vi "dust type.vi"(0 "Enable":bool=TRUE, 1 "Small?":bool, 5 "error in (no error)":errorcluster) -> (14 "Cancel 2":bool caption="Cancel", 15 "output cluster 2":T2 {"Batch" step=1; "Type" step=1; "Dust Source Builder:" items=["Keith Drake", "Nick Beaty", "Anthony Shu", "David James"]}, 16 "Dust Properties 2":T1, 18 "OK":bool, 19 "error out":errorcluster)   [LabVIEW 2012]
doc: "Displays a standard dialog box that prompts users to enter information, such as a user name and password.\n--------------------\n\nThis Express VI is configured as follows:\n\nMessage to Display to the User:Please Enter Experiment Settings Information For Database Storage.\nThe inputs are: \nNumber: Please Enter Group ID\nText Entry Box: Please Enter Tags:\nText Entry Box: Please Enter Experiment Description:"
uses:
  dust type.ctl
  source_builders.ctl
  dust_type_indicator.ctl
  <vilib>/addons/database/Connection.llb/Conn Execute.vi
  <vilib>/addons/database/Recordset.llb/Rec Fetch Recordset Data (R).vi
  <vilib>/addons/database/Recordset.llb/Rec Destroy - Connection.vi
  <userlib>/_OpenG.lib/array/array.llb/Remove Duplicates from 1D Array (String)__ogtk.vi
  <userlib>/_OpenG.lib/array/array.llb/Search 1D Array (String)__ogtk.vi
  <userlib>/_OpenG.lib/array/array.llb/Index 1D Array Elements (I32)__ogtk.vi
  <userlib>/_OpenG.lib/array/array.llb/Conditional Auto-Indexing Tunnel (I32)__ogtk.vi
  <vilib>/addons/database/_DB Variant To Data/Database Variant To Data.xnode
  <vilib>/addons/database/NI_Database_API.lvlib
panel:
  in  "Transfer":bool caption="OK2"
  out "Comments":string[](array[string])
  out "Dust Properties":T1
  out "Dust Names":string[](array[string])
  out "Dust Weights":dbl[](array[numeric])
  out "Sizes":string[](array[string])
  out "Typical Weights":dbl[](array[numeric])
  out "Densities":dbl[](array[numeric])
  out "Batch Nos":i32[](array[numeric])
  out "Dust Types":i32[](array[numeric])
  out "Dust Type Ids":i32[](array[numeric])
  in  "Controls":T2 {"Batch" min=1 max=1 step=1; "Type" min=1 max=2 step=1; "Dust Source Builder:" items=["Keith Drake", "Nick Beaty", "Anthony Shu", "David James"]}
  in  "Create New":bool caption="OK2"
  in  "Cancel":bool
  in  "Update":bool caption="OK1"
  # "Please Enter Dust Information For Storage in the CCLDAS Database."
  # "Dust Information"
  # "Dust Information"
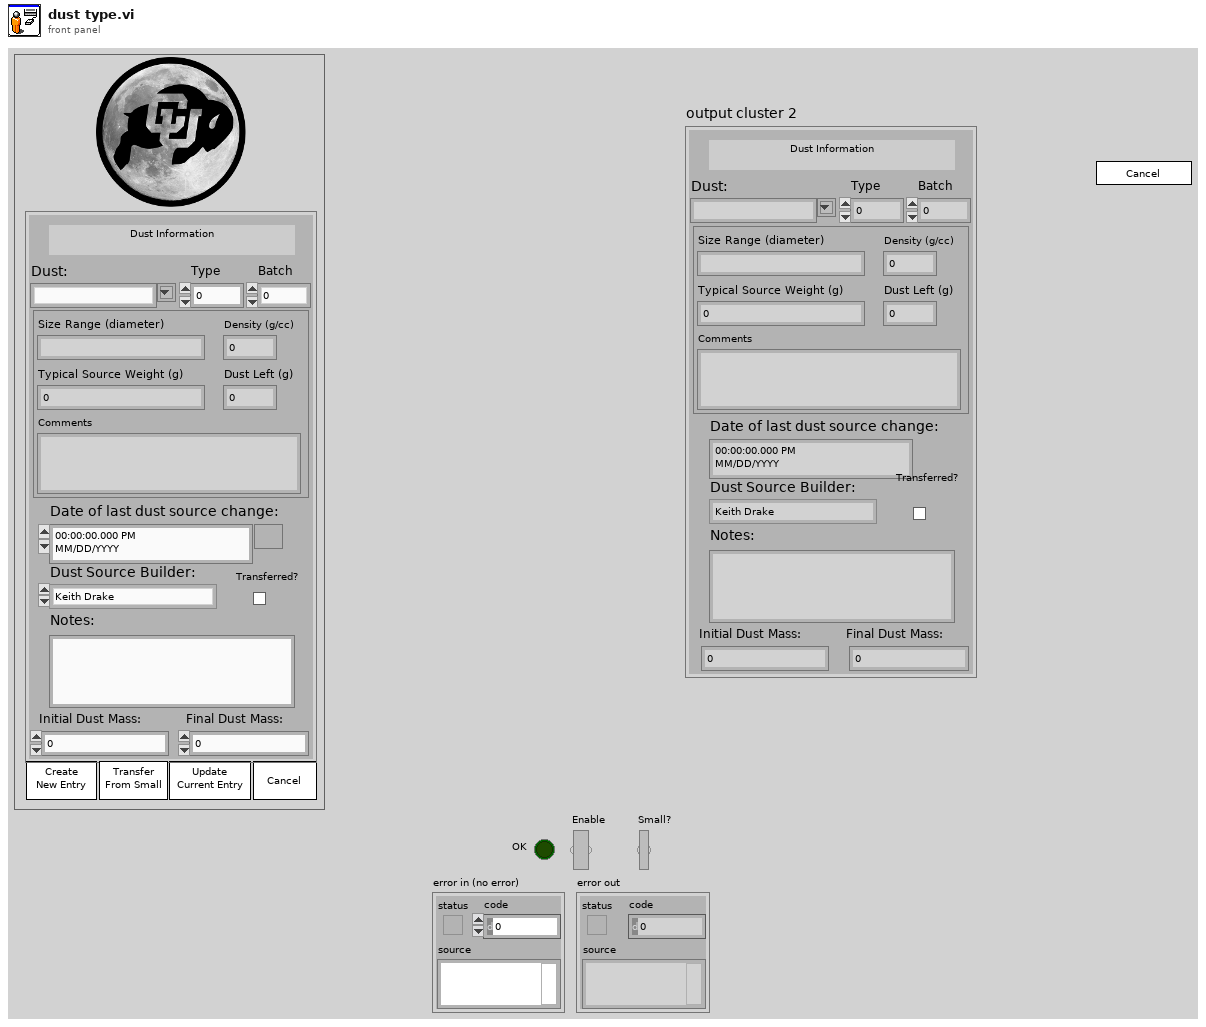
[diagram p1: front panel]
types:
  T1 = typedef "dust_type_indicator.ctl" = cluster{"Size Range (diameter)":string, "Density (g/cc)":dbl, "Typical Source Weight (g)":dbl, "Dust Left (g)":dbl, "Comments":string}
  T2 = typedef "dust type.ctl" = cluster{"Dust info id":u16, "Integer Timestamp":i64, "Dust:":string, "Dust Source Builder:":T3, "Notes:":string, "Date of last dust source change:":timestamp, "Initial Dust Mass:":dbl, "Final Dust Mass:":dbl, "Type":u16, "Batch":u16, "dust type id":u16, "Transferred?":bool}
  T3 = typedef "source_builders.ctl" = u16
  T4 = enum8{"Enabled", "Disabled", "Disabled and Grayed Out"}
  T5 = cluster{"Dust info id":u16, "Integer Timestamp":i64, "dust type id":u16, "Dust Source Builder:":u16, "Notes:":string, "Initial Dust Mass:":dbl, "Final Dust Mass:":dbl, "shot count":u16, "run time":dbl, "From Small\nAccelerator":bool}
  T6 = typedef "NI_Database_API.lvlib/Conn ObjectReference.ctl" = refnum<k1>
  T7 = typedef "NI_Database_API.lvlib/Rec ObjectReference.ctl" = refnum<k1>
  T8 = cluster{"data":string, "data":dbl, "data":dbl, "data":dbl, "data":string}
  T9 = cluster{"Dust event id":dbl, "Integer Time":i64, "dust type id":u16, "Dust Source Builder:":T3, "Notes:":string, "Initial Dust Mass:":dbl, "Dust event id":dbl, "Transferred?":bool}
  T10 = cluster{"Dust event id":dbl, "Integer Time":i64, "dust type id":u16, "Dust Source Builder:":u16, "Notes:":string, "Initial Dust Mass:":dbl, "Final Dust Mass:":dbl, "shot count":u16, "run time":dbl, bool}
  T11 = cluster{"Dust info id":u16, "Integer Timestamp":i64, "dust type id":u16, "Dust Source Builder:":T3, "Notes:":string, "Initial Dust Mass:":dbl, "Final Dust Mass:":dbl, "Transferred?":bool}
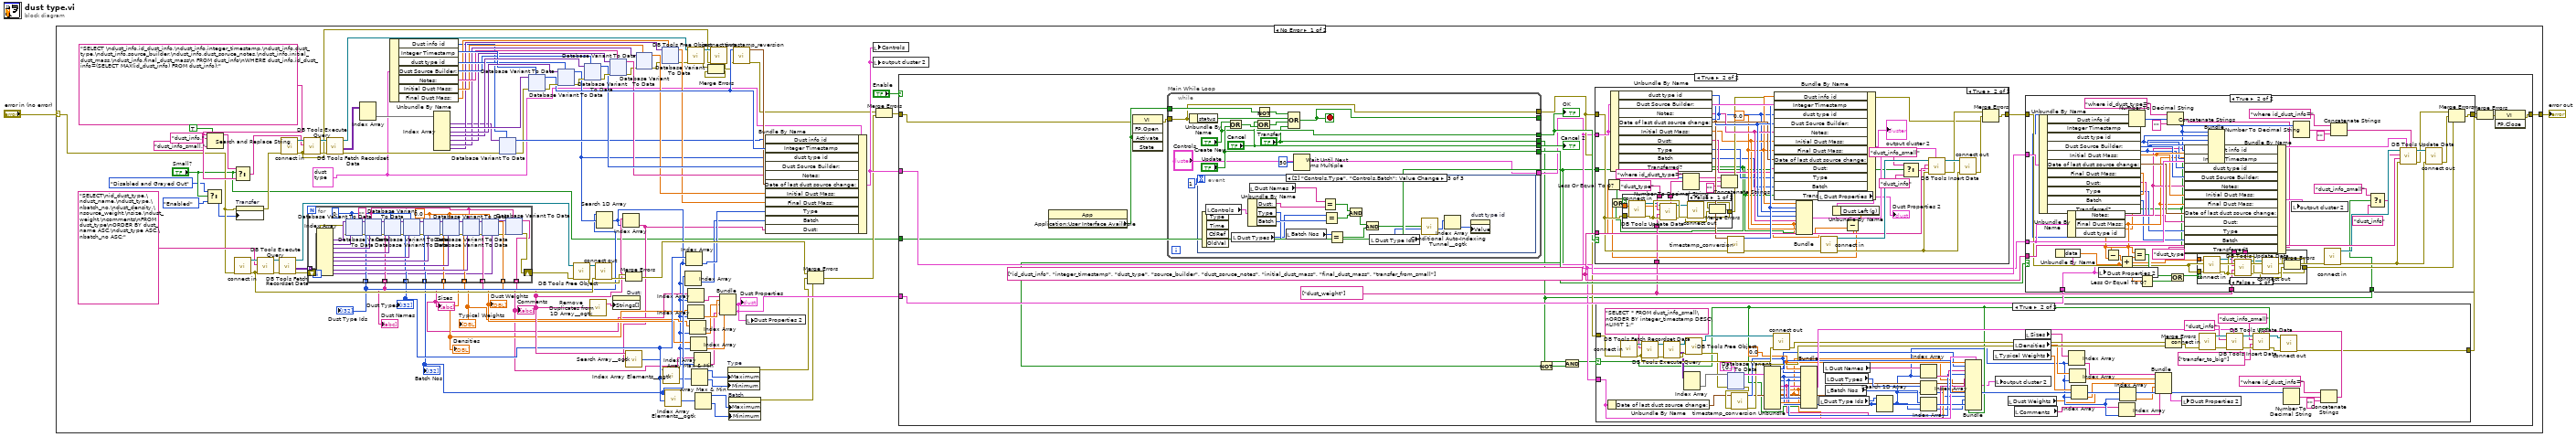
[diagram p0: block diagram]
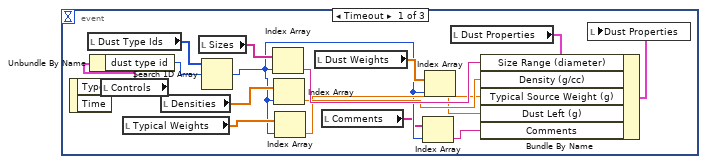
[diagram p6: hidden frame]
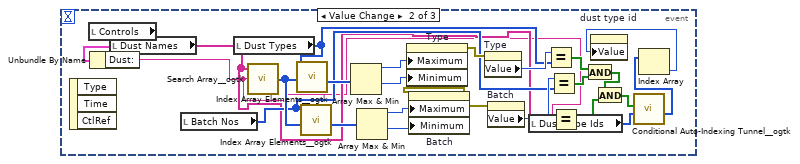
[diagram p7: hidden frame]
diagram:
  n1 = case shown="No Error" "error in (no error)" {
    selector: "error in (no error)" -> [w8 w1234]
    tunnel: [w99 w1234] -> w1
    frame No Error {
      w19 = T2 {"Dust info id"=0, "Integer Timestamp"=0, "Dust:"="", "Dust Source Builder:"=0, "Notes:"="", "Date of last dust source change:"=timestamp(0 s since 1904-01-01), "Initial Dust Mass:"=0.0, "Final Dust Mass:"=0.0, "Type"=0, "Batch"=0, "dust type id"=0, "Transferred?"=FALSE} ("Controls")
      w14 = "SELECT \ndust_info.id_dust_info,\ndust_info.integer_timestamp,\ndust_info.dust_type,\ndust_info.source_builder,\ndust_info.dust_soruce_notes,\ndust_info.initial_dust_mass,\ndust_info.final_dust_mass\n FROM dust_info\nWHERE dust_info.id_dust_info=(SELECT MAX(id_dust_info) FROM dust_info);" ("SQL query")
      n2 = Select(t=T4."Disabled and Grayed Out" ("Disabled"), s="Small?", f=T4."Enabled" ("Disabled")) -> (s? t:f=w3:T4)
      n3 = Search and Replace String(replace all?=TRUE ("replace all? (F)"), input string=w14, search string="dust_info.", replace string="dust_info_small." ("replace string (\"\")")) -> (result string=w13:string)  [unwired: 4 in, 3 out]
      n4 = Select(t=w13, s="Small?", f=w14) -> (s? t:f=w9:string)
      n5 = call "connect in.vi"("error in (no error)"=w8) -> ("error out"=w56:errorcluster, "Database Connection"=w63:T6)  [unwired: 6 in, 1 out]
      n6 = property on="Transfer" class="Bool (strict)"(error in=w8, "DisabledEnum"=w3) -> (error out=w7:errorcluster)  [unwired: 1 in, 1 out]
      n7 = call-poly <vilib>:"DB Tools Execute Query.vi"("error in (no error)"=w56, "SQL query"="SELECT\nid_dust_type,\ndust_name,\ndust_type,\nbatch_no,\ndust_density,\nsource_weight,\nsize,\ndust_weight,\ncomments\nFROM dust_type\nORDER BY dust_name ASC,\ndust_type ASC,\nbatch_no ASC;", "connection reference"=w63) -> ("error out"=w65:errorcluster, "recordset reference"=w64:T7)  [unwired: 5 in]
      n8 = call-poly <vilib>:"DB Tools Fetch Recordset Data.vi"("error in (no error)"=w65, "recordset reference"=w64) -> ("error out"=w60:errorcluster, "recordset data"=w61:variant[][], "recordset reference out"=w57:T7)  [unwired: 3 in]
      n9 = call "connect in.vi"("error in (no error)"=w7) -> ("error out"=w55:errorcluster, "Database Connection"=w100:T6)  [unwired: 6 in, 1 out]
      n10 = call-poly <vilib>:"DB Tools Execute Query.vi"("error in (no error)"=w55, "SQL query"=w9, "connection reference"=w100) -> ("error out"=w102:errorcluster, "recordset reference"=w101:T7)  [unwired: 5 in]
      n11 = for {
        tunnel: w61 -> [w136] mode=indexing
        shift-right: [w106] -> w58
        shift-left: w60 -> [w127]
        tunnel: [w117] -> w48 mode=indexing
        tunnel: [w116] -> w46 mode=indexing
        tunnel: [w115] -> w44 mode=indexing
        tunnel: [w114] -> w43 mode=indexing
        tunnel: [w113] -> w40 mode=indexing
        tunnel: [w112] -> w41 mode=indexing
        tunnel: [w111] -> w39 mode=indexing
        tunnel: [w110] -> w42 mode=indexing
        tunnel: [w105] -> w21 mode=indexing
        w118 = 0.0
        w109 = ""
        w119 = 0
        n12 = Index Array(array=w136) -> (element #1=w135:variant, element #2=w134:variant, element #3=w133:variant, element #4=w132:variant, element #5=w131:variant, element #6=w130:variant, element #7=w129:variant, element #8=w128:variant, element #9=w108:variant)  [unwired: 9 in]
        n13 = xnode "Database Variant To Data"("database variant"=w135, "error in (no error)"=w127, "type"=w119) -> ("data"=w117:i32, "error out"=w126:errorcluster)
        n14 = xnode "Database Variant To Data"("database variant"=w134, "error in (no error)"=w126, "type"=w109) -> ("data"=w116:string, "error out"=w125:errorcluster)
        n15 = xnode "Database Variant To Data"("database variant"=w133, "error in (no error)"=w125, "type"=w119) -> ("data"=w115:i32, "error out"=w124:errorcluster)
        n16 = xnode "Database Variant To Data"("database variant"=w132, "error in (no error)"=w124, "type"=w119) -> ("data"=w114:i32, "error out"=w123:errorcluster)
        n17 = xnode "Database Variant To Data"("database variant"=w131, "error in (no error)"=w123, "type"=w118) -> ("data"=w113:dbl, "error out"=w122:errorcluster)
        n18 = xnode "Database Variant To Data"("database variant"=w130, "error in (no error)"=w122, "type"=w118) -> ("data"=w112:dbl, "error out"=w121:errorcluster)
        n19 = xnode "Database Variant To Data"("database variant"=w129, "error in (no error)"=w121, "type"=w109) -> ("data"=w111:string, "error out"=w120:errorcluster)
        n20 = xnode "Database Variant To Data"("database variant"=w128, "error in (no error)"=w120, "type"=w118) -> ("data"=w110:dbl, "error out"=w107:errorcluster)
        n21 = xnode "Database Variant To Data"("database variant"=w108, "error in (no error)"=w107, "type"=w109) -> ("data"=w105:string, "error out"=w106:errorcluster)
      }
      "Dust Type Ids" <- w48
      "Dust Types" <- w44
      "Batch Nos" <- w43
      "Densities" <- w40
      "Typical Weights" <- w41
      "Sizes" <- w39
      "Dust Weights" <- w42
      "Dust Names" <- w46
      "Comments" <- w21
      n22 = call-poly <vilib>:"DB Tools Fetch Recordset Data.vi"("error in (no error)"=w102, "recordset reference"=w101) -> ("error out"=w67:errorcluster, "recordset data"=w87:variant[][], "recordset reference out"=w103:T7)  [unwired: 3 in]
      n23 = Index Array(array=w87) -> (element=w86:variant[])  [unwired: 2 in]
      n24 = Unbundle By Name(w19) -> ("Dust info id"=w69:u16, "Integer Timestamp"=w93:i64, "dust type id"=w92:u16, "Dust Source Builder:"=w91:T3, "Notes:"=w89:string, "Initial Dust Mass:"=w78:dbl, "Final Dust Mass:"=w76:dbl)
      n25 = Index Array(array=w86) -> (element #1=w70:variant, element #2=w98:variant, element #3=w97:variant, element #4=w95:variant, element #5=w90:variant, element #6=w79:variant, element #7=w74:variant)  [unwired: 7 in]
      n26 = xnode "Database Variant To Data"("database variant"=w70, "error in (no error)"=w67, "type"=w69) -> ("data"=w68:u16, "error out"=w66:errorcluster)
      n27 = xnode "Database Variant To Data"("database variant"=w98, "error in (no error)"=w66, "type"=w93) -> ("data"=w84:i64, "error out"=w96:errorcluster)
      n28 = xnode "Database Variant To Data"("database variant"=w97, "error in (no error)"=w96, "type"=w92) -> ("data"=w49:u16, "error out"=w94:errorcluster)
      n29 = call-poly <vilib>:"DB Tools Free Object.vi"("error in (no error)"=w58, "recordset reference"=w57) -> ("error out"=w50:errorcluster, "connection reference"=w59:T6)  [unwired: 8 in]
      n30 = xnode "Database Variant To Data"("database variant"=w95, "error in (no error)"=w94, "type"=w91) -> ("data"=w81:T3, "error out"=w88:errorcluster)
      n31 = call-poly <userlib>:"Remove Duplicates from 1D Array__ogtk.vi"("Input Array"=w46) -> ("Output Array"=w47:string[])  [unwired: 1 out]
      n32 = call "connect out.vi"("error in (no error)"=w56, "connection reference"=w59) -> ("error out"=w51:errorcluster)  [unwired: 9 in]
      n33 = Search 1D Array(1D array=w48, element=w49) -> (index of element=w22:i32)  [unwired: 1 in]
      n34 = xnode "Database Variant To Data"("database variant"=w90, "error in (no error)"=w88, "type"=w89) -> ("data"=w80:string, "error out"=w73:errorcluster)
      n35 = property on="Dust:" class="CmbBox"("Strings[]"=w47) -> ()  [unwired: 2 in, 2 out]
      n36 = Index Array(array=w46, index=w22) -> (element=w15:string)
      n37 = Merge Errors(w50, w51) -> (w28:errorcluster)
      n38 = call-poly <userlib>:"Search Array__ogtk.vi"("Array"=w46, "Element Data"=w15) -> ("Indices of Elements"=w45:i32[])  [unwired: 7 in]
      n39 = xnode "Database Variant To Data"("database variant"=w79, "error in (no error)"=w73, "type"=w78) -> ("data"=w77:dbl, "error out"=w72:errorcluster)
      n40 = xnode "Database Variant To Data"("database variant"=w74, "error in (no error)"=w72, "type"=w76) -> ("data"=w75:dbl, "error out"=w71:errorcluster)
      n41 = call-poly <userlib>:"Index Array Elements__ogtk.vi"("indices"=w45, "array"=w44) -> ("elements"=w34:i32[])  [unwired: 9 in]
      n42 = call-poly <userlib>:"Index Array Elements__ogtk.vi"("indices"=w45, "array"=w43) -> ("elements"=w33:i32[])  [unwired: 9 in]
      n43 = Index Array(array=w43, index=w22) -> (element=w23:i32)
      n44 = Index Array(array=w44, index=w22) -> (element=w24:i32)
      n45 = call-poly <vilib>:"DB Tools Free Object.vi"("error in (no error)"=w71, "recordset reference"=w103) -> ("error out"=w54:errorcluster, "connection reference"=w104:T6)  [unwired: 8 in]
      n46 = Index Array(array=w39, index=w22) -> (element=w38:string)
      n47 = Index Array(array=w40, index=w22) -> (element=w37:dbl)
      n48 = Index Array(array=w41, index=w22) -> (element=w36:dbl)
      n49 = Index Array(array=w42, index=w22) -> (element=w35:dbl)
      n50 = Array Max & Min(array=w34) -> (max value=w32:i32, min value=w31:i32)  [unwired: 2 out]
      n51 = Index Array(array=w21, index=w22) -> (element=w20:string)
      n52 = Array Max & Min(array=w33) -> (max value=w30:i32, min value=w29:i32)  [unwired: 2 out]
      n53 = call "connect out.vi"("error in (no error)"=w55, "connection reference"=w104) -> ("error out"=w52:errorcluster)  [unwired: 9 in]
      n54 = Merge Errors(w54, w52) -> (w53:errorcluster)
      n55 = Bundle("data"=w38, "data"=w37, "data"=w36, "data"=w35, "data"=w20) -> (w18:T8)  [unwired: 1 in]
      "Dust Properties" <- w18
      n56 = property on="Type" class="DigNum (strict)"("Maximum"=w32, "Minimum"=w31) -> (error out=w17:errorcluster)  [unwired: 2 in, 1 out]
      n57 = property on="Batch" class="DigNum (strict)"("Maximum"=w30, "Minimum"=w29) -> (error out=w16:errorcluster)  [unwired: 2 in, 1 out]
      n58 = call "timestamp_reversion.vi"("error in (no error)"=w53, "Integer Timestamp"=w84) -> ("error out"=w26:errorcluster, "time stamp"=w82:timestamp)  [unwired: 7 in]
      n59 = local write "Dust Properties 2"(w18) -> ()
      n60 = Bundle By Name(cluster=w19, "Dust info id"=w68, "Integer Timestamp"=w84, "dust type id"=w49, "Dust Source Builder:"=w81, "Notes:"=w80, "Date of last dust source change:"=w82, "Initial Dust Mass:"=w77, "Final Dust Mass:"=w75, "Type"=w24, "Batch"=w23, "Dust:"=w15) -> (w83:T2)
      n61 = Merge Errors(w28, w17, w16) -> (w25:errorcluster)
      n62 = local write "Controls"(w83) -> ()
      n63 = local write "output cluster 2"(w83) -> ()
      n64 = Merge Errors(w26, w25) -> (w27:errorcluster)
      n65 = case shown="True" "Enable" {
        tunnel: w27 -> [w521 w526]
        tunnel: [w521 w541] -> w99
        tunnel: w83 -> [_ w536]
        tunnel: w18 -> [_ w533]
        tunnel: "Small?" -> [_ w524]
        frame False {
        }
        frame True {
          w534 = string[] ["dust_weight"]
          w537 = string[] ["id_dust_info", "integer_timestamp", "dust_type", "source_builder", "dust_soruce_notes", "initial_dust_mass", "final_dust_mass", "transfer_from_small"] ("columns")
          n66 = property class="App"() -> ("Application:User Interface Available"=w535:bool)  [unwired: 2 in, 2 out]
          n67 = invoke class="VI" method="FP.Open"(error in=w526, "Activate"=w535) -> (error out=w542:errorcluster)  [unwired: 3 in, 4 out]
          n68 = while "Main While Loop" {
            tunnel: w535 -> [w996]
            tunnel: [w992] -> _
            tunnel: w542 -> [w990]
            tunnel: [w990] -> w531
            tunnel: ["Cancel"] -> w540
            tunnel: ["Controls"] -> w530
            tunnel: ["Update"] -> w539
            tunnel: ["Create New"] -> w532
            tunnel: ["Transfer"] -> w522
            stop <- w992 stop-if-true
            n69 = Unbundle By Name(w990) -> ("status"=w993:bool)
            n70 = event shown="[2] \"Controls.Type\", \"Controls.Batch\": Value Change" {
              selector: _ -> [_ _ _]
              dyn-events: _ -> [_ _ _]
              timeout: 1 -> [_ _ _]
              event Timeout {
                n71 = event-data() -> ()  [unwired: 1 in, 2 out]
                n72 = local read "Dust Type Ids"() -> (w1013:i32[])
                n73 = local read "Controls"() -> (w999:T2)
                n74 = Unbundle By Name(w999) -> ("dust type id"=w1014:u16)
                n75 = local read "Typical Weights"() -> (w1010:dbl[])
                n76 = local read "Densities"() -> (w1011:dbl[])
                n77 = local read "Sizes"() -> (w1012:string[])
                n78 = Search 1D Array(1D array=w1013, element=w1014) -> (index of element=w1002:i32)  [unwired: 1 in]
                n79 = Index Array(array=w1012, index=w1002) -> (element=w1006:string)
                n80 = Index Array(array=w1011, index=w1002) -> (element=w1005:dbl)
                n81 = Index Array(array=w1010, index=w1002) -> (element=w1004:dbl)
                n82 = local read "Dust Weights"() -> (w1009:dbl[])
                n83 = local read "Comments"() -> (w1001:string[])
                n84 = Index Array(array=w1001, index=w1002) -> (element=w1000:string)
                n85 = Index Array(array=w1009, index=w1002) -> (element=w1003:dbl)
                n86 = local read "Dust Properties"() -> (w1007:T1)
                n87 = Bundle By Name(cluster=w1007, "Size Range (diameter)"=w1006, "Density (g/cc)"=w1005, "Typical Source Weight (g)"=w1004, "Dust Left (g)"=w1003, "Comments"=w1000) -> (w1008:T1)
                n88 = local write "Dust Properties"(w1008) -> ()
              }
              event Value Change {
                n89 = event-data() -> ()  [unwired: 1 in, 3 out]
                n90 = local read "Controls"() -> (w1016:T2)
                n91 = Unbundle By Name(w1016) -> ("Dust:"=w1015:string)
                n92 = local read "Dust Names"() -> (w1025:string[])
                n93 = local read "Batch Nos"() -> (w1026:i32[])
                n94 = local read "Dust Types"() -> (w1028:i32[])
                n95 = call-poly <userlib>:"Search Array__ogtk.vi"("Array"=w1025, "Element Data"=w1015) -> ("Indices of Elements"=w1037:i32[])  [unwired: 7 in]
                n96 = call-poly <userlib>:"Index Array Elements__ogtk.vi"("indices"=w1037, "array"=w1028) -> ("elements"=w1036:i32[])  [unwired: 9 in]
                n97 = call-poly <userlib>:"Index Array Elements__ogtk.vi"("indices"=w1037, "array"=w1026) -> ("elements"=w1038:i32[])  [unwired: 9 in]
                n98 = Array Max & Min(array=w1036) -> (max value=w1035:i32, min value=w1034:i32)  [unwired: 2 out]
                n99 = Array Max & Min(array=w1038) -> (max value=w1033:i32, min value=w1032:i32)  [unwired: 2 out]
                n100 = property on="Type" class="DigNum (strict)"("Maximum"=w1035, "Minimum"=w1034) -> (error out=w1031:errorcluster)  [unwired: 2 in, 1 out]
                n101 = property on="Batch" class="DigNum (strict)"("Maximum"=w1033, "Minimum"=w1032) -> (error out=w1030:errorcluster)  [unwired: 2 in, 1 out]
                n102 = property on="Type" class="DigNum (strict)"(error in=w1031) -> ("Value"=w1029:u16)  [unwired: 1 in, 2 out]
                n103 = property on="Batch" class="DigNum (strict)"(error in=w1030) -> ("Value"=w1027:u16)  [unwired: 1 in, 2 out]
                n104 = local read "Dust Type Ids"() -> (w1019:i32[])
                n105 = Equal?(x=w1029, y=w1028) -> (x = y?=w1024:bool[])
                n106 = Equal?(x=w1027, y=w1026) -> (x = y?=w1023:bool[])
                n107 = Equal?(x=w1015, y=w1025) -> (x = y?=w1021:bool[])
                n108 = And(x=w1024, y=w1023) -> (x .and. y?=w1022:bool[])
                n109 = And(x=w1022, y=w1021) -> (x .and. y?=w1020:bool[])
                n110 = call-poly <userlib>:"Conditional Auto-Indexing Tunnel__ogtk.vi"("Array in"=w1019, "Elements to keep"=w1020) -> ("Filtered Array out"=w1018:i32[])  [unwired: 5 in]
                n111 = Index Array(array=w1018) -> (element=w1017:i32)  [unwired: 1 in]
                n112 = property on="dust type id" class="Ring (strict)"("Value"=w1017) -> ()  [unwired: 2 in, 2 out]
              }
              event Value Change {
                n113 = event-data() -> ()  [unwired: 1 in, 4 out]
                n114 = local read "Controls"() -> (w1040:T2)
                n115 = local read "Dust Types"() -> (w1049:i32[])
                n116 = Unbundle By Name(w1040) -> ("Dust:"=w1039:string, "Type"=w1053:u16, "Batch"=w1052:u16)
                n117 = local read "Dust Names"() -> (w1051:string[])
                n118 = local read "Batch Nos"() -> (w1050:i32[])
                n119 = Equal?(x=w1051, y=w1039) -> (x = y?=w1048:bool[])
                n120 = Equal?(x=w1049, y=w1053) -> (x = y?=w1047:bool[])
                n121 = Equal?(x=w1050, y=w1052) -> (x = y?=w1045:bool[])
                n122 = And(x=w1048, y=w1047) -> (x .and. y?=w1046:bool[])
                n123 = And(x=w1046, y=w1045) -> (x .and. y?=w1044:bool[])
                n124 = local read "Dust Type Ids"() -> (w1043:i32[])
                n125 = call-poly <userlib>:"Conditional Auto-Indexing Tunnel__ogtk.vi"("Array in"=w1043, "Elements to keep"=w1044) -> ("Filtered Array out"=w1042:i32[])  [unwired: 5 in]
                n126 = Index Array(array=w1042) -> (element=w1041:i32)  [unwired: 1 in]
                n127 = property on="dust type id" class="Ring (strict)"("Value"=w1041) -> ()  [unwired: 2 in, 2 out]
              }
            }
            n128 = Or(x="Create New", y="Update") -> (x .or. y?=w997:bool)
            n129 = Or(x="Cancel", y=w997) -> (x .or. y?=w994:bool)
            n130 = Not(x=w996) -> (.not. x?=w995:bool)
            n131 = Compound Arithmetic op=OR(w995, w993, w994, "Transfer") -> (w992:bool)
            n132 = Wait Until Next ms Multiple(millisecond multiple=u32 50) -> ()  [unwired: 1 out]
          }
          "OK" <- w532
          "Cancel 2" <- w540
          n133 = Not(x=w524) -> (.not. x?=w523:bool)
          n134 = And(x=w522, y=w523) -> (x .and. y?=w525:bool)
          n135 = case shown="True" w532 {
            tunnel: w531 -> [w1054 w1077]
            tunnel: [w1054 w1081] -> w538
            tunnel: w530 -> [_ w1087]
            tunnel: w537 -> [_ w1080]
            tunnel: w534 -> [_ w1075]
            tunnel: w524 -> [_ w1056]
            frame False {
            }
            frame True {
              w1078 = 0.0 ("Dust event id")
              n136 = Unbundle By Name(w1087) -> ("dust type id"=w1064:u16, "Dust Source Builder:"=w1084:T3, "Notes:"=w1083:string, "Date of last dust source change:"=w1079:timestamp, "Initial Dust Mass:"=w1072:dbl, "Dust:"=w1063:string, "Type"=w1062:u16, "Batch"=w1061:u16, "Transferred?"=w1059:bool)
              n137 = Number To Decimal String(number=w1064) -> (decimal integer string=w1067:string)  [unwired: 1 in]
              n138 = Concatenate Strings("where id_dust_type=" ("condition"), w1067, "" ("string")) -> (w1065:string)
              n139 = call "timestamp_conversion.vi"("error in (no error)"=w1077, "Time Stamp"=w1079) -> ("error out"=w1093:errorcluster, "Integer Time"=w1085:i64)  [unwired: 7 in]
              n140 = Bundle By Name(cluster=w1087, "Dust info id"=w1078, "Integer Timestamp"=w1085, "dust type id"=w1064, "Dust Source Builder:"=w1084, "Notes:"=w1083, "Initial Dust Mass:"=w1072, "Final Dust Mass:"=w1078, "Date of last dust source change:"=w1079, "Dust:"=w1063, "Type"=w1062, "Batch"=w1061, "Transferred?"=w1059) -> (→"output cluster 2":T2)
              n141 = Bundle("Dust event id"=w1078, "Integer Time"=w1085, "dust type id"=w1064, "Dust Source Builder:"=w1084, "Notes:"=w1083, "Initial Dust Mass:"=w1072, "Dust event id"=w1078, "Transferred?"=w1059) -> (w1082:T9)  [unwired: 1 in]
              n142 = local read "Dust Properties"() -> (w1073:T1)
              "Dust Properties 2" <- w1073
              n143 = call "connect in.vi"("error in (no error)"=w1093) -> ("error out"=w1090:errorcluster, "Database Connection"=w1092:T6)  [unwired: 6 in, 1 out]
              n144 = Unbundle By Name(w1073) -> ("Dust Left (g)"=w1069:dbl)
              n145 = Less Or Equal To 0?(x=w1069) -> (x <= 0?=w1070:bool)
              n146 = Or(x=w1070, y=w1059) -> (x .or. y?=w1060:bool)
              n147 = Subtract(x=w1069, y=w1072) -> (x-y=w1071:dbl)
              n148 = case shown="False" w1060 {
                tunnel: [w1101 w1105] -> w1076
                tunnel: w1077 -> [w1100 w1105]
                tunnel: w1075 -> [w1099 _]
                tunnel: "dust_type" -> [w1098 _]
                tunnel: w1071 -> [w1095 _]
                tunnel: w1065 -> [w1094 _]
                frame False {
                  n149 = call "connect in.vi"("error in (no error)"=w1100) -> ("error out"=w1104:errorcluster, "Database Connection"=w1097:T6)  [unwired: 6 in, 1 out]
                  n150 = call <vilib>:"DB Tools Update Data.vi"("condition"=w1094, "data"=w1095, "error in (no error)"=w1104, "columns"=w1099, "table"=w1098, "connection reference"=w1097) -> ("error out"=w1103:errorcluster, "connection reference out"=w1096:T6)  [unwired: 4 in]
                  n151 = call "connect out.vi"("error in (no error)"=w1104, "connection reference"=w1096) -> ("error out"=w1102:errorcluster)  [unwired: 9 in]
                  n152 = Merge Errors(w1102, w1103) -> (w1101:errorcluster)
                }
                frame True {
                }
              }
              n153 = Select(t="dust_info_small" ("table"), s=w1056, f="dust_info" ("table")) -> (s? t:f=w1055:string)
              n154 = call <vilib>:"DB Tools Insert Data.vi"("data"=w1082, "error in (no error)"=w1090, "columns"=w1080, "table"=w1055, "connection reference"=w1092) -> ("error out"=w1089:errorcluster, "connection reference out"=w1091:T6)  [unwired: 5 in]
              n155 = call "connect out.vi"("error in (no error)"=w1090, "connection reference"=w1091) -> ("error out"=w1088:errorcluster)  [unwired: 9 in]
              n156 = Merge Errors(w1089, w1088, w1076) -> (w1081:errorcluster)
            }
          }
          n157 = case shown="True" w525 {
            selector: w525 -> [_ w557]
            tunnel: w531 -> [w543 w607]
            tunnel: w530 -> [_ w573]
            tunnel: [w543 w574] -> w527
            frame False {
            }
            frame True {
              w572 = 0.0 ("Dust event id")
              n158 = Unbundle By Name(w573) -> ("Date of last dust source change:"=w562:timestamp)
              n159 = call "connect in.vi"("error in (no error)"=w607) -> ("error out"=w605:errorcluster, "Database Connection"=w606:T6)  [unwired: 6 in, 1 out]
              n160 = call-poly <vilib>:"DB Tools Execute Query.vi"("error in (no error)"=w605, "SQL query"="SELECT * FROM dust_info_small\nORDER BY integer_timestamp DESC\nLIMIT 1;", "connection reference"=w606) -> ("error out"=w609:errorcluster, "recordset reference"=w608:T7)  [unwired: 5 in]
              n161 = call-poly <vilib>:"DB Tools Fetch Recordset Data.vi"("error in (no error)"=w609, "recordset reference"=w608) -> ("error out"=w603:errorcluster, "recordset data"=w600:variant[][], "recordset reference out"=w604:T7)  [unwired: 3 in]
              n162 = Index Array(array=w600) -> (element=w599:variant[])  [unwired: 2 in]
              n163 = call-poly <vilib>:"DB Tools Free Object.vi"("error in (no error)"=w603, "recordset reference"=w604) -> ("error out"=w598:errorcluster, "connection reference"=w602:T6)  [unwired: 8 in]
              n164 = xnode "Database Variant To Data"("database variant"=w599, "error in (no error)"=w598, "type"=T5 {"Dust info id"=0, "Integer Timestamp"=0, "dust type id"=0, "Dust Source Builder:"=0, "Notes:"="", "Initial Dust Mass:"=0.0, "Final Dust Mass:"=0.0, "shot count"=0, "run time"=0.0, "From Small\nAccelerator"=FALSE}) -> ("data"=w594:T5, "error out"=w589:errorcluster)
              n165 = call "timestamp_conversion.vi"("error in (no error)"=w589, "Time Stamp"=w562) -> ("error out"=w576:errorcluster, "Integer Time"=w571:i64)  [unwired: 7 in]
              n166 = Unbundle(w594) -> ("Dust info id"=w581:u16, "dust type id"=w570:u16, "Dust Source Builder:"=w564:u16, "Notes:"=w563:string, "Initial Dust Mass:"=w561:dbl, "Final Dust Mass:"=w560:dbl, "shot count"=w592:u16, "run time"=w591:dbl)  [unwired: 2 out]
              n167 = call "connect out.vi"("error in (no error)"=w605, "connection reference"=w602) -> ("error out"=w577:errorcluster)  [unwired: 9 in]
              n168 = Bundle("Dust event id"=w572, "Integer Time"=w571, "dust type id"=w570, "Dust Source Builder:"=w564, "Notes:"=w563, "Initial Dust Mass:"=w561, "Final Dust Mass:"=w560, "shot count"=w592, "run time"=w591, w557) -> (w590:T10)  [unwired: 1 in]
              n169 = local read "Dust Type Ids"() -> (w569:i32[])
              n170 = local read "Dust Names"() -> (w568:string[])
              n171 = local read "Dust Types"() -> (w567:i32[])
              n172 = local read "Batch Nos"() -> (w566:i32[])
              n173 = Search 1D Array(1D array=w569, element=w570) -> (index of element=w549:i32)  [unwired: 1 in]
              n174 = Index Array(array=w568, index=w549) -> (element=w565:string)
              n175 = Index Array(array=w567, index=w549) -> (element=w559:i32)
              n176 = Index Array(array=w566, index=w549) -> (element=w558:i32)
              n177 = Bundle(cluster=w573, "Dust info id"=w572, "Integer Timestamp"=w571, "Dust:"=w565, "Dust Source Builder:"=w564, "Notes:"=w563, "Date of last dust source change:"=w562, "Initial Dust Mass:"=w561, "Final Dust Mass:"=w560, "Type"=w559, "Batch"=w558, "dust type id"=w570, "Transferred?"=w557) -> (w556:T2)
              n178 = local read "Typical Weights"() -> (w553:dbl[])
              n179 = local write "output cluster 2"(w556) -> ()
              n180 = local read "Dust Weights"() -> (w548:dbl[])
              n181 = local read "Densities"() -> (w554:dbl[])
              n182 = local read "Comments"() -> (w547:string[])
              n183 = local read "Sizes"() -> (w555:string[])
              n184 = Index Array(array=w555, index=w549) -> (element=w552:string)
              n185 = Index Array(array=w554, index=w549) -> (element=w551:dbl)
              n186 = Index Array(array=w553, index=w549) -> (element=w550:dbl)
              n187 = Index Array(array=w547, index=w549) -> (element=w545:string)
              n188 = Index Array(array=w548, index=w549) -> (element=w546:dbl)
              n189 = Bundle("data"=w552, "data"=w551, "data"=w550, "data"=w546, "data"=w545) -> (w544:T8)  [unwired: 1 in]
              n190 = Merge Errors(w577, w576) -> (w575:errorcluster)
              n191 = local write "Dust Properties 2"(w544) -> ()
              n192 = call "connect in.vi"("error in (no error)"=w575) -> ("error out"=w596:errorcluster, "Database Connection"=w597:T6)  [unwired: 6 in, 1 out]
              n193 = call <vilib>:"DB Tools Insert Data.vi"("data"=w590, "error in (no error)"=w596, "table"="dust_info", "connection reference"=w597) -> ("error out"=w586:errorcluster, "connection reference out"=w588:T6)  [unwired: 6 in]
              n194 = Number To Decimal String(number=w581) -> (decimal integer string=w583:string)  [unwired: 1 in]
              n195 = Concatenate Strings("where id_dust_info=" ("condition"), w583, "" ("string")) -> (w580:string)
              n196 = call <vilib>:"DB Tools Update Data.vi"("condition"=w580, "data"=w557, "error in (no error)"=w586, "columns"=string[] ["transfer_to_big"], "table"="dust_info_small", "connection reference"=w588) -> ("error out"=w579:errorcluster, "connection reference out"=w578:T6)  [unwired: 4 in]
              n197 = call "connect out.vi"("error in (no error)"=w579, "connection reference"=w578) -> ("error out"=w574:errorcluster)  [unwired: 9 in]
            }
          }
          n198 = case shown="True" w539 {
            tunnel: [w924 w966] -> w528
            tunnel: w538 -> [w924 w948]
            tunnel: w537 -> [_ w972]
            tunnel: w530 -> [_ w959]
            tunnel: w536 -> [_ w960]
            tunnel: w534 -> [_ w947]
            tunnel: w533 -> [_ w930]
            tunnel: w522 -> [_ w927]
            frame False {
            }
            frame True {
              n199 = Unbundle By Name(w960) -> ("Dust info id"=w954:u16, "Integer Timestamp"=w955:i64, "dust type id"=w956:u16, "Dust Source Builder:"=w957:T3, "Initial Dust Mass:"=w958:dbl, "Date of last dust source change:"=w953:timestamp, "Final Dust Mass:"=w943:dbl, "Dust:"=w933:string, "Type"=w932:u16, "Batch"=w931:u16, "Transferred?"=w929:bool)
              n200 = Unbundle By Name(w930) -> ("data"=w935:dbl)
              n201 = Unbundle By Name(w959) -> ("Notes:"=w951:string, "Final Dust Mass:"=w945:dbl, "dust type id"=w938:u16)
              n202 = local write "Dust Properties 2"(w930) -> ()
              n203 = Subtract(x=w945, y=w943) -> (x-y=w944:dbl)
              n204 = Add(x=w944, y=w935) -> (x+y=w942:dbl)
              n205 = Number To Decimal String(number=w938) -> (decimal integer string=w940:string)  [unwired: 1 in]
              n206 = Equal?(x=w943, y=w945) -> (x = y?=w950:bool)
              n207 = Less Or Equal To 0?(x=w935) -> (x <= 0?=w934:bool)
              n208 = Concatenate Strings("where id_dust_type=" ("condition"), w940, "" ("string")) -> (w937:string)
              n209 = Or(x=w950, y=w934) -> (x .or. y?=w936:bool)
              n210 = Bundle By Name(cluster=w959, "Dust info id"=w954, "Integer Timestamp"=w955, "dust type id"=w956, "Dust Source Builder:"=w957, "Notes:"=w951, "Initial Dust Mass:"=w958, "Final Dust Mass:"=w945, "Date of last dust source change:"=w953, "Dust:"=w933, "Type"=w932, "Batch"=w931, "Transferred?"=w929) -> (w961:T2)
              n211 = case shown="False" w936 {
                tunnel: [w980 w984] -> w949
                tunnel: w948 -> [w979 w984]
                tunnel: w947 -> [w978 _]
                tunnel: "dust_type" -> [w977 _]
                tunnel: w942 -> [w974 _]
                tunnel: w937 -> [w973 _]
                frame False {
                  n212 = call "connect in.vi"("error in (no error)"=w979) -> ("error out"=w983:errorcluster, "Database Connection"=w976:T6)  [unwired: 6 in, 1 out]
                  n213 = call <vilib>:"DB Tools Update Data.vi"("condition"=w973, "data"=w974, "error in (no error)"=w983, "columns"=w978, "table"=w977, "connection reference"=w976) -> ("error out"=w982:errorcluster, "connection reference out"=w975:T6)  [unwired: 4 in]
                  n214 = call "connect out.vi"("error in (no error)"=w983, "connection reference"=w975) -> ("error out"=w981:errorcluster)  [unwired: 9 in]
                  n215 = Merge Errors(w981, w982) -> (w980:errorcluster)
                }
                frame True {
                }
              }
              n216 = Bundle("Dust info id"=w954, "Integer Timestamp"=w955, "dust type id"=w956, "Dust Source Builder:"=w957, "Notes:"=w951, "Initial Dust Mass:"=w958, "Final Dust Mass:"=w945, "Transferred?"=w929) -> (w952:T11)  [unwired: 1 in]
              n217 = local write "output cluster 2"(w961) -> ()
              n218 = Number To Decimal String(number=w954) -> (decimal integer string=w964:string)  [unwired: 1 in]
              n219 = call "connect in.vi"("error in (no error)"=w948) -> ("error out"=w967:errorcluster, "Database Connection"=w971:T6)  [unwired: 6 in, 1 out]
              n220 = Concatenate Strings("where id_dust_info=" ("condition"), w964, "" ("string")) -> (w962:string)
              n221 = Select(t="dust_info_small" ("table"), s=w927, f="dust_info" ("table")) -> (s? t:f=w926:string)
              n222 = call <vilib>:"DB Tools Update Data.vi"("condition"=w962, "data"=w952, "error in (no error)"=w967, "columns"=w972, "table"=w926, "connection reference"=w971) -> ("error out"=w969:errorcluster, "connection reference out"=w970:T6)  [unwired: 4 in]
              n223 = call "connect out.vi"("error in (no error)"=w967, "connection reference"=w970) -> ("error out"=w968:errorcluster)  [unwired: 9 in]
              n224 = Merge Errors(w969, w968, w949) -> (w966:errorcluster)
            }
          }
          n225 = Merge Errors(w528, w527) -> (w529:errorcluster)
          n226 = invoke class="VI" method="FP.Close"(error in=w529) -> (error out=w541:errorcluster)  [unwired: 2 in, 2 out]
        }
      }
    }
    frame Error {
    }
  }
  "error out" <- w1
